vi "FSR.vi"() -> ()   [LabVIEW 2018]
panel:
  out "Force Reached":bool
  out "Force":dbl
  out "Force":dbl(graph)
  in  "stop (F)":bool
  # "Using 10k ohm Rm value"
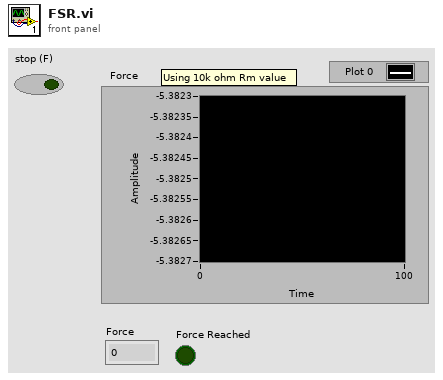
[diagram p1: front panel]
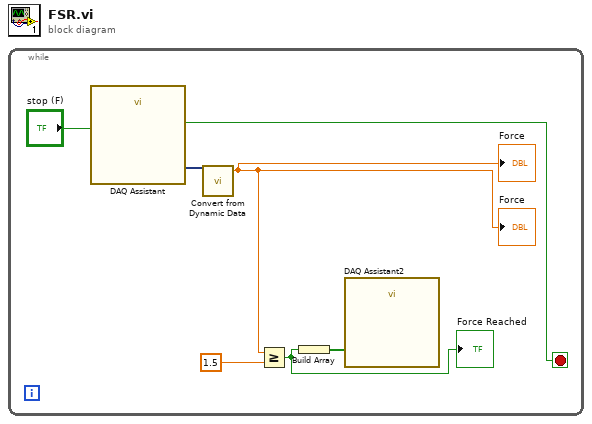
[diagram p0: block diagram]
diagram:
  n1 = while {
    stop <- w6 stop-if-true
    n2 = call "DAQ Assistant"("stop (F)"="stop (F)") -> ("data"=w5:dynamicdata, "stopped"=w6:bool)  [unwired: 15 in, 2 out]
    n3 = call "Convert from Dynamic Data"("Dynamic Data Type"=w5) -> ("Scalar"=w1:dbl)  [unwired: 3 in]
    "Force" <- w1
    "Force" <- w1
    n4 = Greater Or Equal?(x=w1, y=1.5) -> (x >= y?=w3:bool)
    "Force Reached" <- w3
    n5 = Build Array(w3) -> (w2:bool[])
    n6 = call "DAQ Assistant2"("data"=w2) -> ()  [unwired: 17 in, 2 out]
  }
